vi "Test Set Subpanels-- Config-- Error Generation.vi"(8 "error in":errorcluster) -> (0 "error out":errorcluster)   [LabVIEW 2019]
uses:
  Maui 2.0/Maui 2.0.lvclass
  C:/Program Files (x86)/National Instruments/LabVIEW 2019/vi.lib/JKI/JKI SMO/SMO/SMO.lvclass
  Maui 2.0/Typedefs/Maui 2.0/Maui 2.0 Configuration.ctl
  <vilib>/addons/_JKI Toolkits/Caraya/classes/Assert/Assert Error.vi
  <vilib>/addons/_JKI Toolkits/Caraya/classes/Assert/Assert True.vi
  <vilib>/JKI/JKI SMO/SMO/SMO.lvclass
  <vilib>/Utility/config.llb/NI_LVConfig.lvlib
  <vilib>/addons/_JKI Toolkits/Caraya/classes/Test/Test.lvclass
  <vilib>/addons/_JKI Toolkits/Caraya/classes/Assert/Assert.lvclass
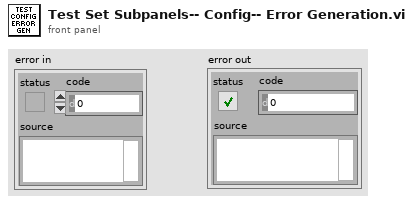
[diagram p1: front panel]
types:
  T1 = typedef "Maui 2.0.lvclass/Maui 2.0 Configuration.ctl" = cluster{"Paths":path[]}
  T2 = typedef "NI_LVConfig.lvlib/Config Data RefNum.ctl" = refnum<k1>
  T3 = cluster{"Subpanels":T1, "Extraneous":cluster{path[], i32}}
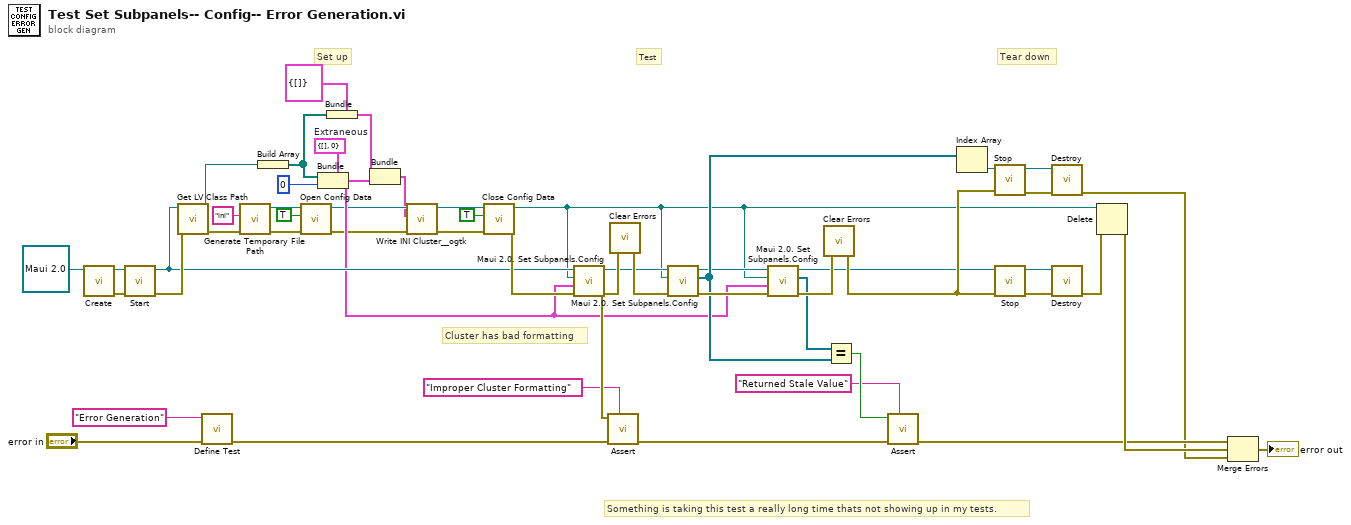
[diagram p0: block diagram]
diagram:
  w21 = cluster{path[], i32} {[], 0}  # Extraneous
  # "Cluster has bad formatting"
  # "Something is taking this test a really long time thats not showing up in my tests."
  # "Tear down"
  # "Test"
  # "Set up"
  n1 = call <vilib>:"Create.vi"("SMO"=refnum<class "Maui 2.0.lvclass"> refnum ("Maui 2.0.lvclass")) -> ("error out"=w52:errorcluster, "SMO out"=w31:refnum<class "Maui 2.0.lvclass">)  [unwired: 8 in, 1 out]
  n2 = call <vilib>:"Start.vi"("error in (no error)"=w52, "SMO"=w31) -> ("error out"=w50:errorcluster, "SMO out"=w27:refnum<class "Maui 2.0.lvclass">)  [unwired: 8 in]
  n3 = call <vilib>:"Get LV Class Path.vi"("error in (no error)"=w50, "object"=w27) -> ("error out"=w45:errorcluster, "class path"=w25:path)  [unwired: 8 in]
  n4 = call <vilib>:"Define Test.vi"("error in (no error)"="error in", "Label (VI Title)"="Error Generation") -> ("error out"=w42:errorcluster)  [unwired: 9 in]
  n5 = call <vilib>:"Generate Temporary File Path.vi"("error in (no error)"=w45, "Temporary File Extension (tmp)"="ini") -> ("error out"=w44:errorcluster, "Unique Temporary File Path"=w23:path)  [unwired: 8 in]
  n6 = Build Array(w25) -> (w19:path[])
  n7 = call <vilib>:"Open Config Data.vi"("error in (no error)"=w44, "create file if necessary (T)"=TRUE, "configuration file path"=w23) -> ("error out"=w3:errorcluster, "refnum"=w5:T2)  [unwired: 6 in, 1 out]
  n8 = Bundle(cluster=w21, w19, 0) -> (w7:cluster{path[], i32})
  n9 = Bundle(cluster=T1 {"Paths"=[]} ("Subpanels"), "Paths"=w19) -> (w6:T1)
  n10 = Bundle("Subpanels"=w6, "Extraneous"=w7) -> (w1:T3)  [unwired: 1 in]
  n11 = call <userlib>:"Write INI Cluster__ogtk.vi"("error in (no error)"=w3, "INI Fomatted Cluster"=w1, "refnum"=w5) -> ("error out"=w2:errorcluster, "dup refnum"=w4:T2)  [unwired: 7 in]
  n12 = call <vilib>:"Close Config Data.vi"("error in (no error)"=w2, "write file if changed (T)"=TRUE, "refnum"=w4) -> ("error out"=w49:errorcluster, "file path"=w9:path)  [unwired: 7 in]
  n13 = call-dynamic "Maui 2.0. Set Subpanels.Config.vi"("error in"=w49, "Section Cluster"=w7, "Path"=w9, "Maui 2.0 in"=w27) -> ("error out"=w34:errorcluster, "Maui 2.0 out"=w17:refnum<class "Maui 2.0.lvclass">)  [unwired: 4 in, 2 out]
  n14 = call-poly <vilib>:"Assert.vi"("Label"="Improper Cluster Formatting", "error in (no error)"=w42, "Error?"=w34) -> ("error out"=w40:errorcluster)  [unwired: 8 in]
  n15 = call <vilib>:"Clear Errors.vi"("error in (no error)"=w34) -> ("error out"=w41:errorcluster)  [unwired: 5 in, 1 out]
  n16 = call-dynamic "Maui 2.0. Set Subpanels.Config.vi"("error in"=w41, "Path"=w9, "Maui 2.0 in"=w17) -> ("error out"=w36:errorcluster, "Subpanels"=w12:refnum<class "SMO.lvclass">[], "Maui 2.0 out"=w10:refnum<class "Maui 2.0.lvclass">)  [unwired: 5 in, 1 out]
  n17 = call-dynamic "Maui 2.0. Set Subpanels.Config.vi"("error in"=w36, "Section Cluster"=w7, "Path"=w9, "Maui 2.0 in"=w10) -> ("error out"=w35:errorcluster, "Subpanels"=w16:refnum<class "SMO.lvclass">[], "Maui 2.0 out"=w8:refnum<class "Maui 2.0.lvclass">)  [unwired: 4 in, 1 out]
  n18 = call <vilib>:"Clear Errors.vi"("error in (no error)"=w35) -> ("error out"=w33:errorcluster)  [unwired: 5 in, 1 out]
  n19 = Equal?(x=w16, y=w12) -> (x = y?=w15:bool)
  n20 = call-poly <vilib>:"Assert.vi"("Label"="Returned Stale Value", "error in (no error)"=w40, "True?"=w15) -> ("error out"=w39:errorcluster)  [unwired: 8 in]
  n21 = Index Array(array=w12) -> (element=w11:refnum<class "SMO.lvclass">)  [unwired: 1 in]
  n22 = call <vilib>:"Stop.vi"("error in (no error)"=w33, "SMO"=w11) -> ("error out"=w38:errorcluster, "SMO out"=w13:refnum<class "SMO.lvclass">)  [unwired: 8 in]
  n23 = call <vilib>:"Stop.vi"("error in (no error)"=w33, "SMO"=w8) -> ("error out"=w51:errorcluster, "SMO out"=w30:refnum<class "Maui 2.0.lvclass">)  [unwired: 8 in]
  n24 = call <vilib>:"Destroy.vi"("error in (no error)"=w38, "SMO"=w13) -> ("error out"=w37:errorcluster)  [unwired: 9 in]
  n25 = call <vilib>:"Destroy.vi"("error in (no error)"=w51, "SMO"=w30) -> ("error out"=w46:errorcluster)  [unwired: 9 in]
  n26 = Delete(path (use dialog)=w9, error in=w46) -> (error out=w43:errorcluster)  [unwired: 3 in, 2 out]
  n27 = Merge Errors(w39, w43, w37) -> (→"error out":errorcluster)
